vi "DAQ state machine with subvi.vi"() -> ()   [LabVIEW 2017]
uses:
  <vilib>/OPCUA/controls/Write Status.ctl
  <vilib>/OPCUA/controls/NodeId.ctl
  <vilib>/OPCUA/NI OPC UA Client.lvlib
  <vilib>/OPCUA/client/Multiple Write Double.vi
  <vilib>/OPCUA/client/Multiple Write Bool.vi
  <vilib>/OPCUA/controls/Subscription ID.ctl
  <vilib>/OPCUA/controls/OPC UA StatusCode.ctl
  <vilib>/OPCUA/controls/OPC UA Client Refnum.ctl
  <vilib>/OPCUA/controls/Subscription Data Change.ctl
  <vilib>/OPCUA/controls/Data Type.ctl
  <vilib>/OPCUA/controls/NodeIds.ctl
panel:
  out "Number of Disconnections":u32
  out "Available Elements for Reading":i32
  out "DAQ?":bool
  out "error out":errorcluster
  in  "error in (no error)":errorcluster
  out "Connection Status":bool
  in  "Stop":bool
  in  "Disconnect":bool
  in  "Connect to Server":bool
  in  "Flow Data?":bool=TRUE
  in  "Power Output On":bool
  in  "CTAH Set Point":sgl format="%.1f"
  in  "Pump Frequency [Hz]":dbl min=0.0 max=45.0 step=0.10000000149011612 format="%.1f"
  in  "Desired Power [W]":dbl min=0.0 max=10000.0 step=1.0 format="%.1f"
  in  "TCHX Frequency [Hz]":dbl min=0.0 max=60.0 step=0.10000000149011612 format="%.1f"
  out "Frequency [Hz] 3":dbl(slide) scale=0.0..60.0
  out "Frequency [Hz]":dbl(knob) scale=0.0..45.0
  out "WT-67":dbl format="%.1f"
  out "WT-64":dbl format="%.1f"
  out "WT-62":dbl format="%.1f"
  out "WT-61":dbl format="%.1f"
  out "WT-42":dbl format="%.1f"
  out "WT-40":dbl format="%.1f"
  out "WT-35":dbl format="%.1f"
  out "WT-33":dbl format="%.1f"
  out "WT-31":dbl format="%.1f"
  out "WT-28":dbl format="%.1f"
  out "WT-26":dbl format="%.1f"
  out "WT-24":dbl format="%.1f"
  out "WT-22":dbl format="%.1f"
  out "WT-20":dbl format="%.1f"
  out "WT-13":dbl format="%.1f"
  out "WT-10":dbl format="%.1f"
  out "ST-14w":dbl format="%.1f"
  out "ST-14s":dbl format="%.1f"
  out "ST-14n":dbl format="%.1f"
  out "ST-14e":dbl format="%.1f"
  out "ST-13":dbl format="%.1f"
  out "ST-12sw":dbl format="%.1f"
  out "ST-12se":dbl format="%.1f"
  out "ST-12n":dbl format="%.1f"
  out "ST-11":dbl format="%.1f"
  out "ST-10":dbl format="%.1f"
  out "CX-114":dbl format="%.1f"
  out "CX-113":dbl format="%.1f"
  out "CX-112":dbl format="%.1f"
  out "CX-111":dbl format="%.1f"
  out "CX-104":dbl format="%.1f"
  out "CX-103":dbl format="%.1f"
  out "CX-102":dbl format="%.1f"
  out "CX-101":dbl format="%.1f"
  out "BT-66":dbl format="%.1f"
  out "BT-65":sgl format="%.1f"
  out "BT-63":dbl format="%.1f"
  out "BT-60":dbl format="%.1f"
  out "BT-43":dbl format="%.1f"
  out "BT-41":dbl format="%.1f"
  out "BT-34":dbl format="%.1f"
  out "BT-32":dbl format="%.1f"
  out "BT-30":dbl format="%.1f"
  out "BT-29":sgl format="%.1f"
  out "BT-27":dbl format="%.1f"
  out "BT-25":dbl format="%.1f"
  out "BT-23":dbl format="%.1f"
  out "BT-21":dbl format="%.1f"
  out "BT-12":dbl format="%.1f"
  out "BT-11":dbl format="%.1f"
  out "20001":dbl
  out "AT-02":dbl format="%.1f"
  out "AT-01":dbl format="%.1f"
  out "System Time":timestamp
  out "DRACS Flow\n\n\nFM-60 [kg/s]":dbl format="%.3f"
  out "Primary Flow\n\n\nFM-40 [kg/s]":dbl format="%.3f"
  out "Bypass Flow\n\n\nFM-30 [kg/s]":dbl format="%.3f"
  out "DHX Primary Flow\n\n\nFM-20 [kg/s]":dbl format="%.3f"
  out "Temperature":dbl
  out "Time Stamp 2":timestamp
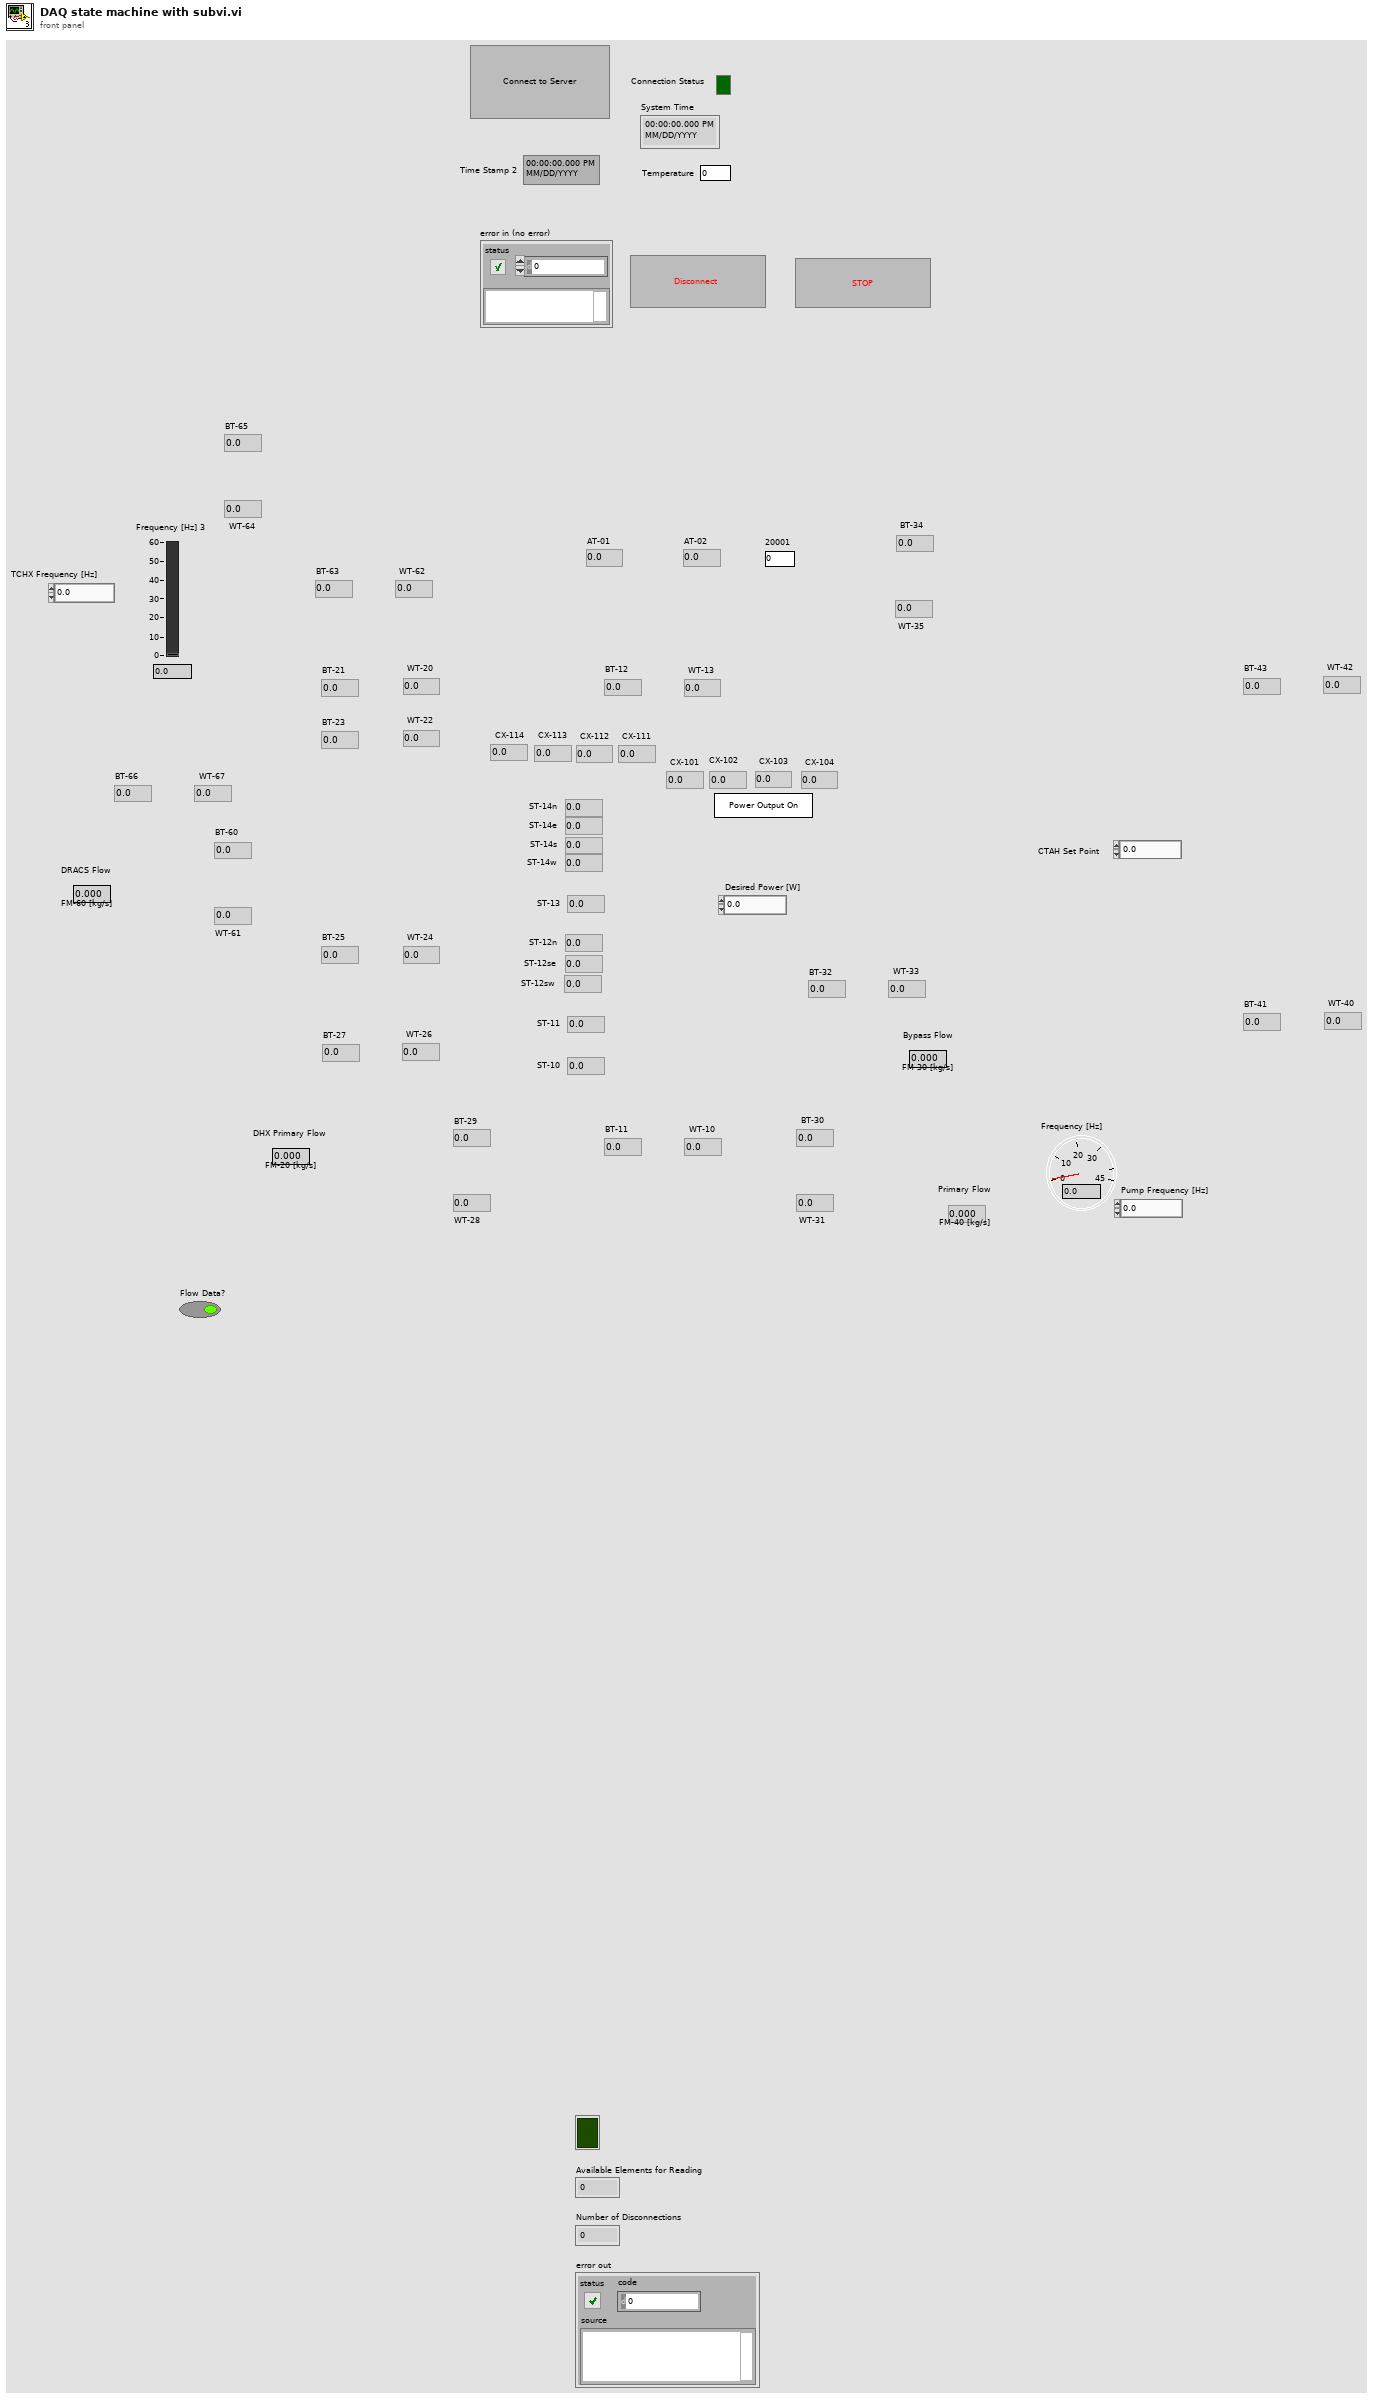
[diagram p1: front panel]
types:
  T1 = typedef "NodeId.ctl" = string
  T2 = typedef "Write Status.ctl" = u32
  T3 = cluster{"node ID":T1, "value":dbl, "timestamp (current time)":timestamp, "node status":T2}
  T4 = cluster{"node ID":T1, "value":bool, "timestamp (current time)":timestamp, "node status":T2}
  T5 = cluster{"message mode":enum16{"None", "Sign", "Sign and Encrypt"}, "security":enum16{"Basic256", "Basic128Rsa15"}}
  T6 = typedef "OPC UA Client Refnum.ctl" = refnum<k21>
  T7 = typedef "Subscription Data Change.ctl" = cluster{"node ID":T1, " value":variant, "timestamp":timestamp, "data type":T8, "status code":T9}
  T8 = typedef "Data Type.ctl" = u16
  T9 = typedef "OPC UA StatusCode.ctl" = u32
  T10 = cluster{"node ID":T1, "value":dbl, "timestamp (current time)":timestamp, "node status":T2}[]
  T11 = cluster{"node ID":T1, "value":bool, "timestamp (current time)":timestamp, "node status":T2}[]
  T12 = typedef "Subscription ID.ctl" = u32
  T13 = cluster{"OPC UA Data Change Event Registration Refnum":refnum<event-registration>, "OPC UA client refnum ":T6, "OPC UA Subscription Service Status":T9, "OPC UA Subscription ID":T12, "OPC UA Monitored Nodes":string[], "Connection Status":bool}
  T14 = typedef "NodeIds.ctl" = T1[]
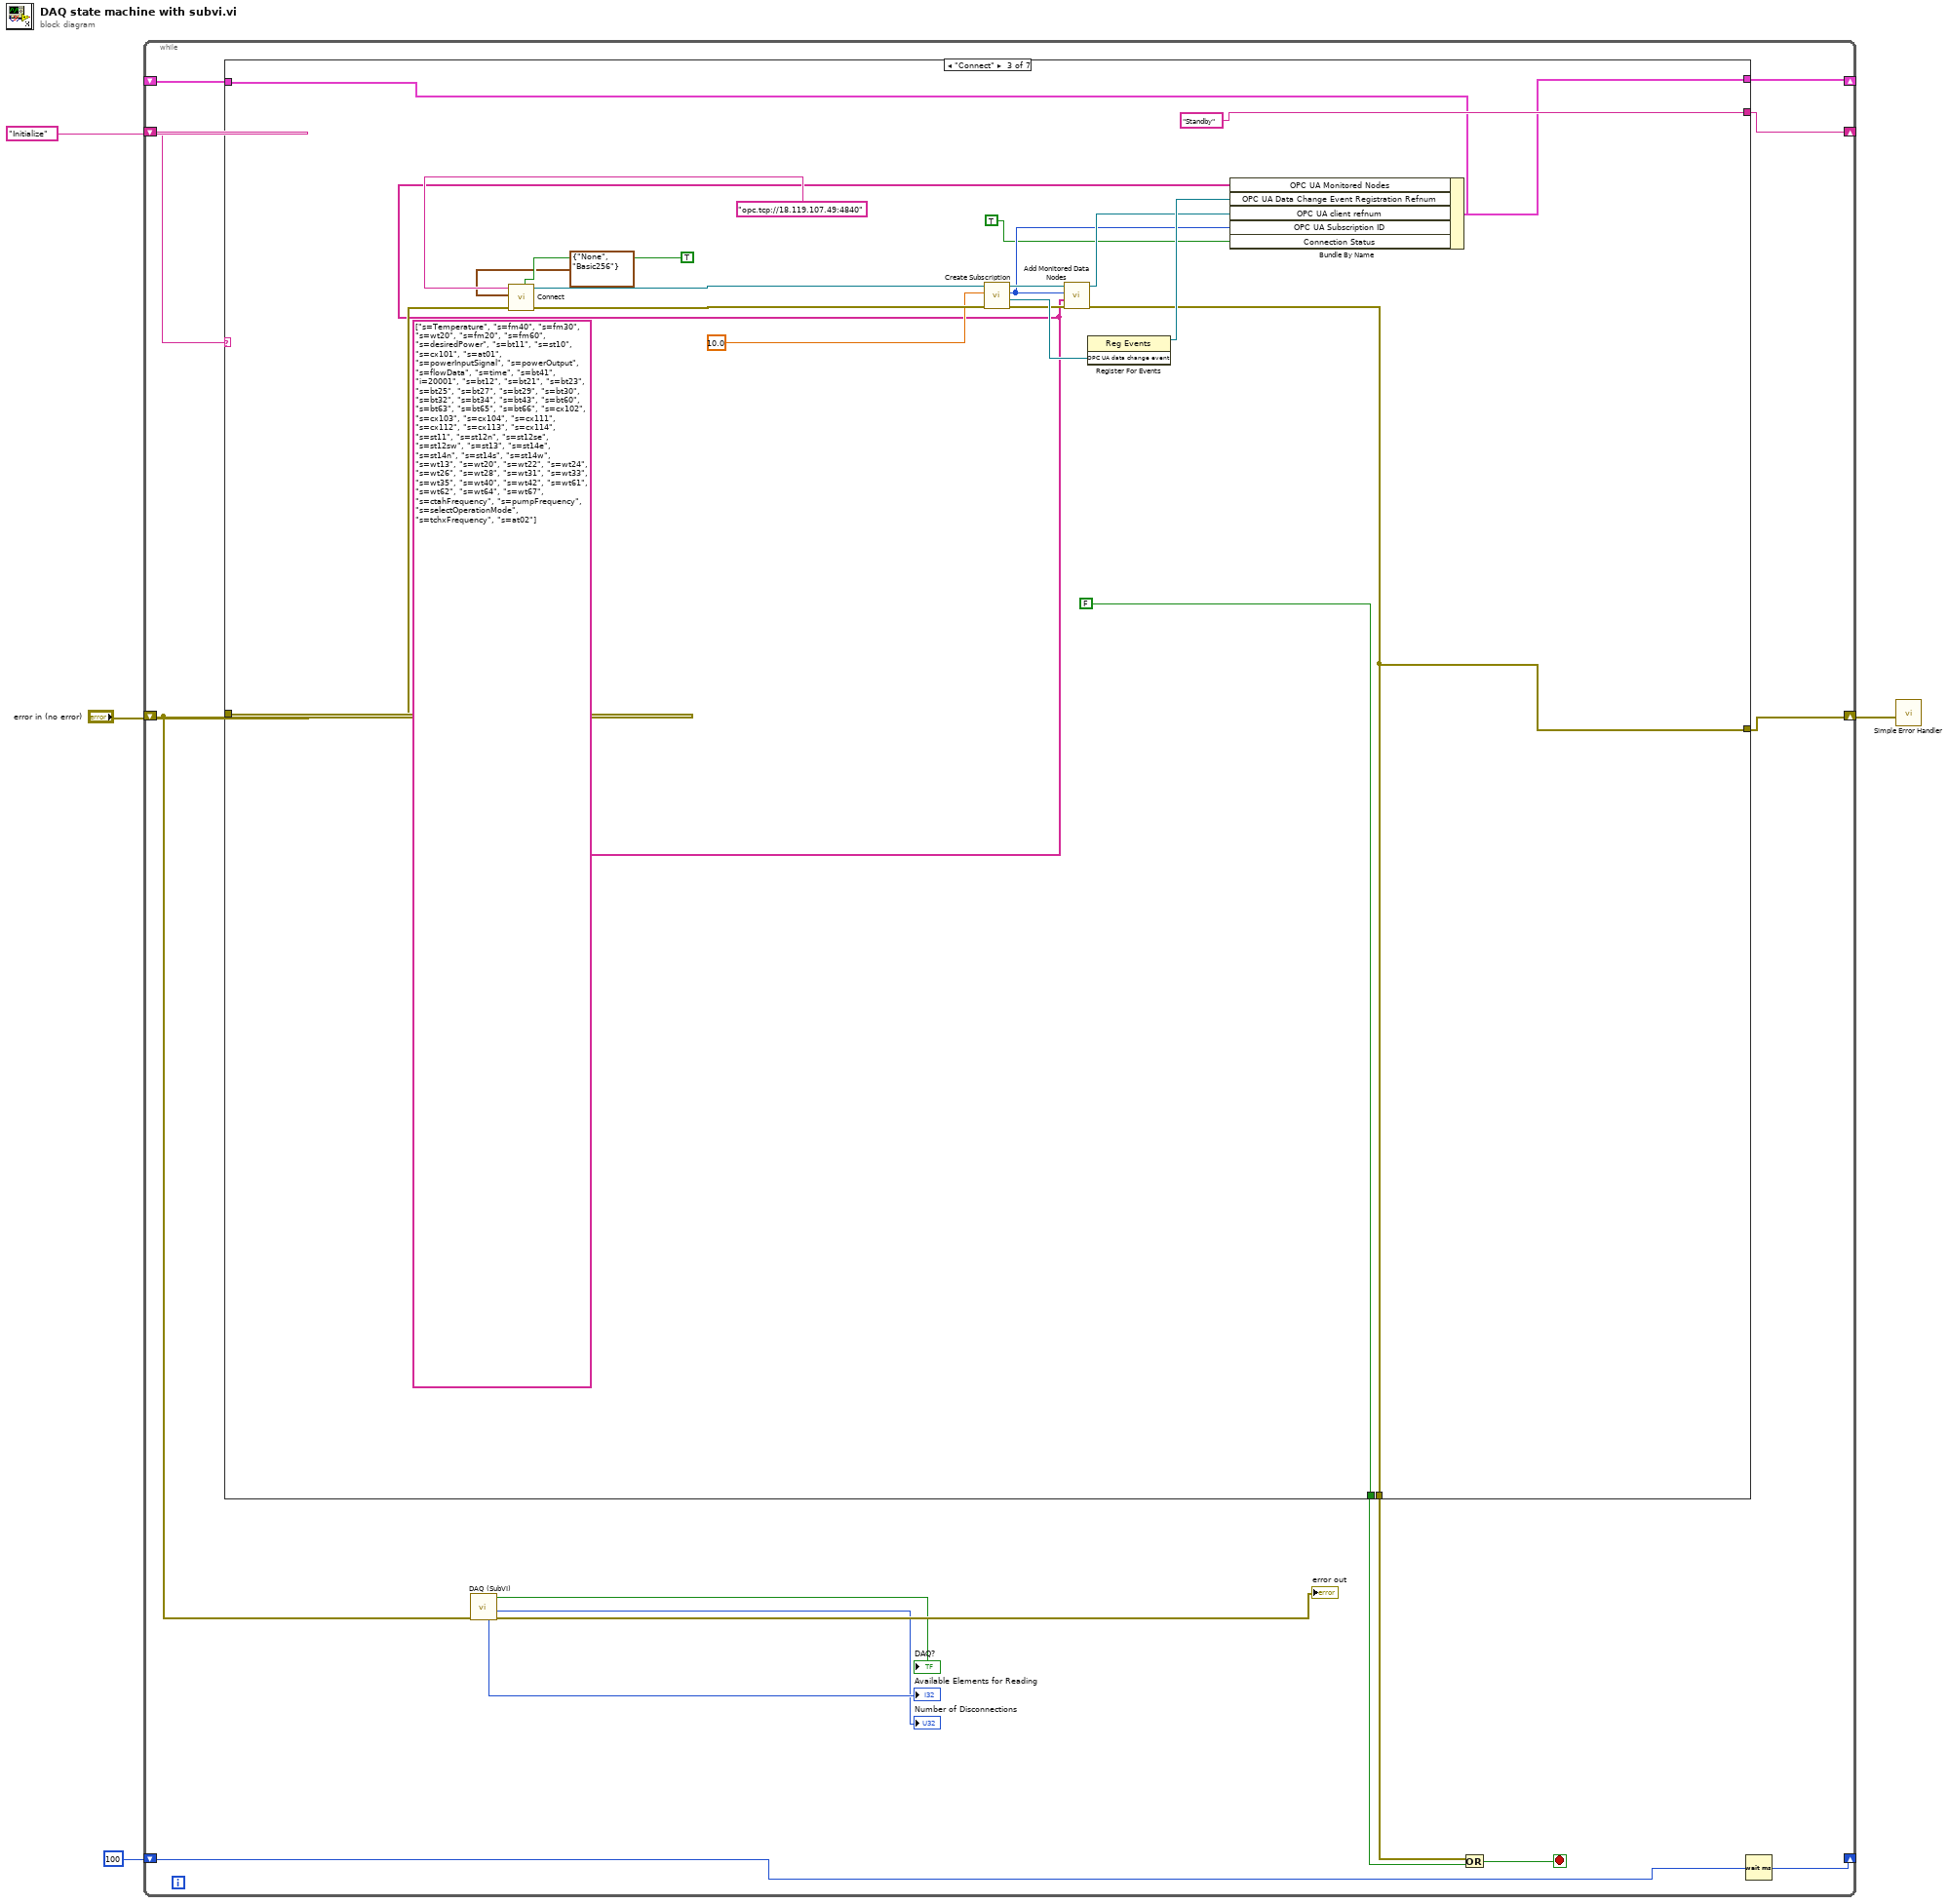
[diagram p0: block diagram]
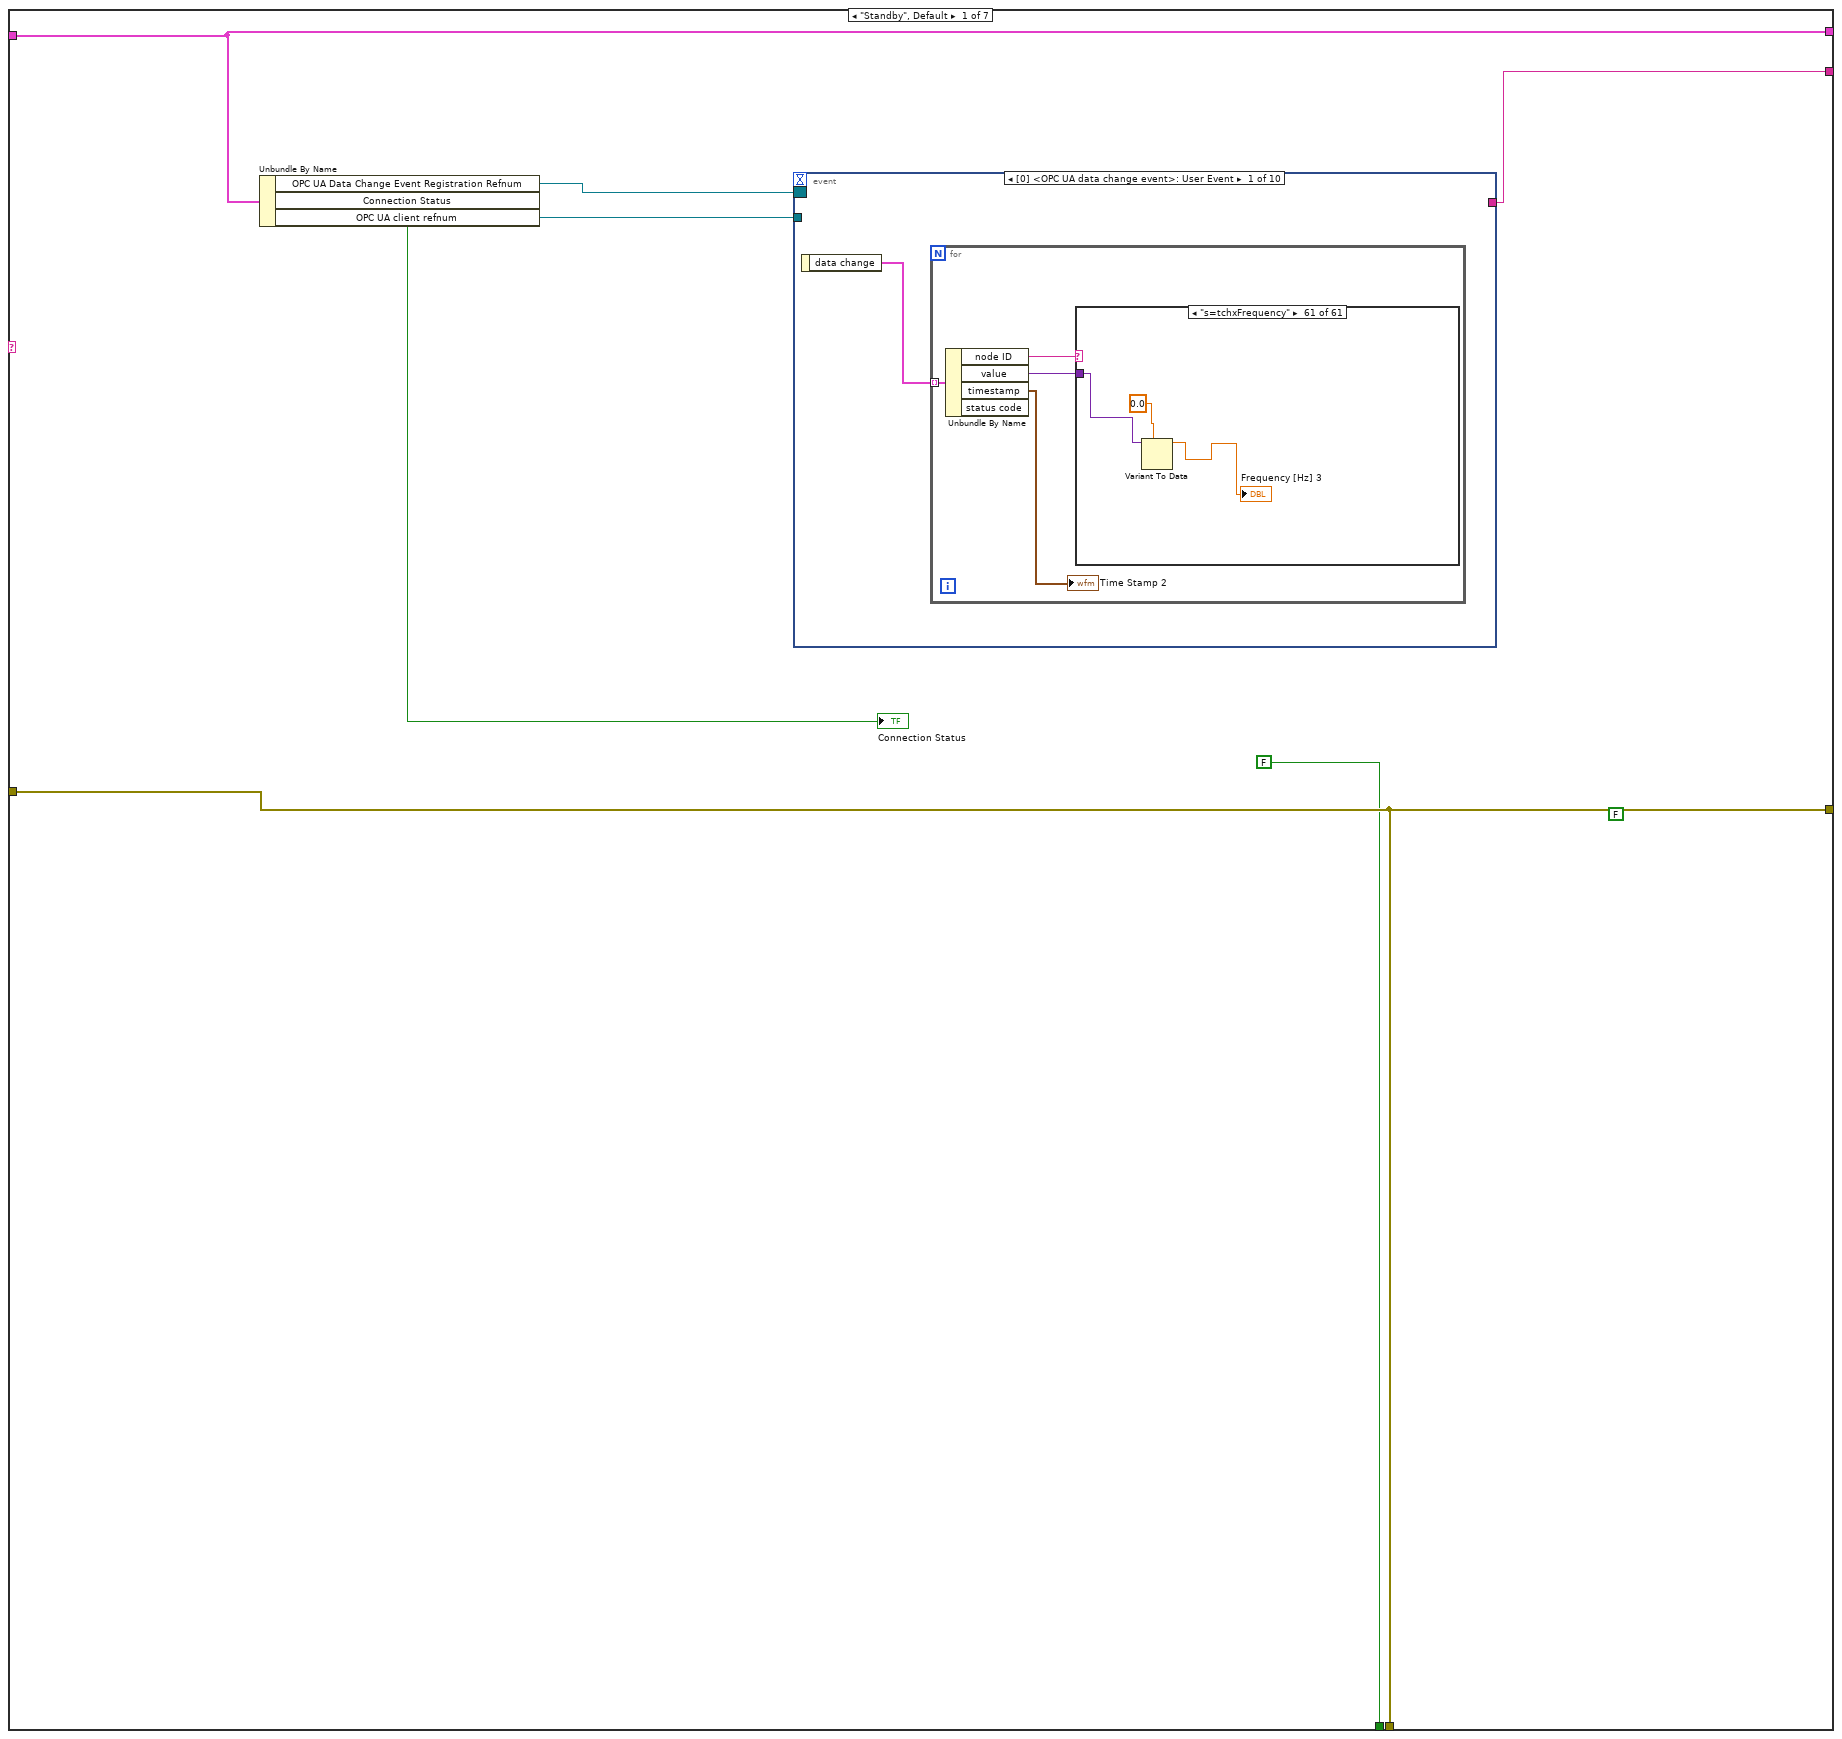
[diagram p2: hidden frame]
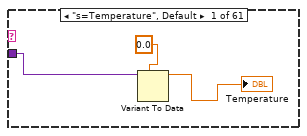
[diagram p3: hidden frame]
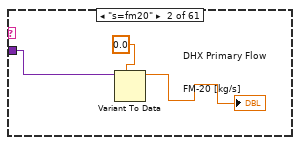
[diagram p4: hidden frame]
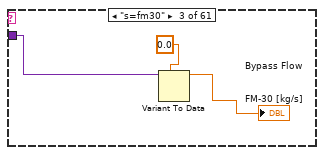
[diagram p5: hidden frame]
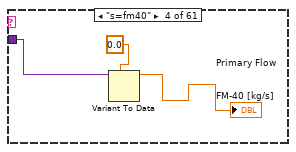
[diagram p6: hidden frame]
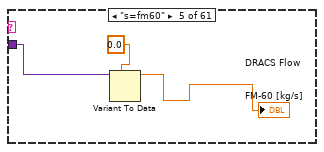
[diagram p7: hidden frame]
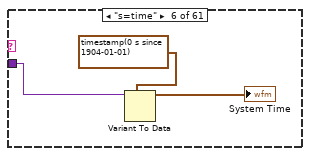
[diagram p8: hidden frame]
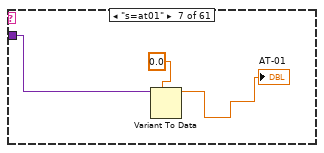
[diagram p9: hidden frame]
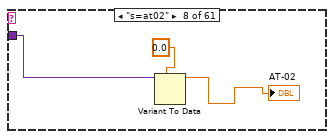
[diagram p10: hidden frame]
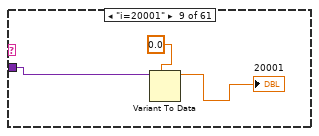
[diagram p11: hidden frame]
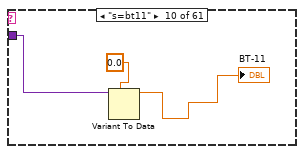
[diagram p12: hidden frame]
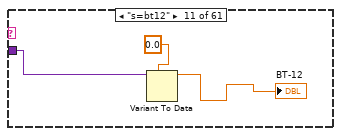
[diagram p13: hidden frame]
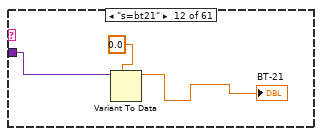
[diagram p14: hidden frame]
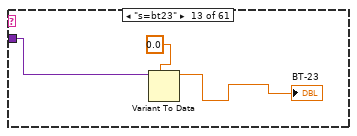
[diagram p15: hidden frame]
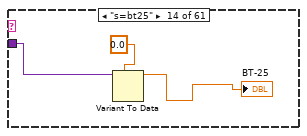
[diagram p16: hidden frame]
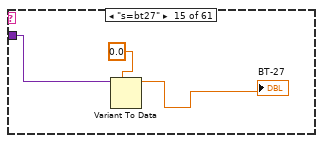
[diagram p17: hidden frame]
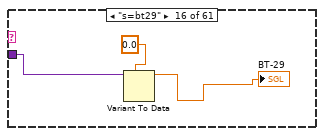
[diagram p18: hidden frame]
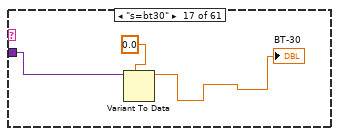
[diagram p19: hidden frame]
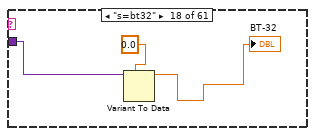
[diagram p20: hidden frame]
diagram:
  n1 = while {
    shift-right: [w15] -> _
    shift-left: _ -> [w16]
    shift-right: [w14] -> w3
    shift-left: "error in (no error)" -> [w5]
    shift-right: [w12] -> _
    shift-left: "Initialize" -> [w13]
    shift-right: [w10] -> _
    shift-left: u32 100 ("millisecond timer value") -> [w11]
    stop <- w18 stop-if-true
    n2 = case shown="\"Connect\"" w13 {
      tunnel: w5 -> [w22 w267 w285 w299 w318 w333 w342]
      tunnel: [w22 w267 w279 w299 w313 w328 w342] -> w19
      tunnel: [FALSE FALSE FALSE FALSE FALSE FALSE TRUE] -> w17
      tunnel: [w24 "Standby" "Standby" w300 "Standby" "Stop" "Initialize"] -> w12
      tunnel: [w23 w269 w278 w298 w311 w326 w341] -> w15
      tunnel: w16 -> [w23 w268 w281 w298 w312 w327 w341]
      tunnel: [w22 w267 w279 w299 w313 w328 w342] -> w14
      frame "Standby", Default {
        (unwired) FALSE
        n3 = Unbundle By Name(w23) -> ("OPC UA Data Change Event Registration Refnum"=w25:refnum<event-registration>, "Connection Status"=→"Connection Status":bool, "OPC UA client refnum"=w20:T6)
        n4 = event shown="[0] <OPC UA data change event>: User Event" {
          selector: w25 -> [_ _ _ _ _ _ _ _ _ _]
          dyn-events: _ -> [_ _ _ _ _ _ _ _ _ _]
          timeout: _ -> [_ _ _ _ _ _ _ _ _ _]
          tunnel: [_ _ _ _ _ _ _ "Connect" "Disconnect" "Stop Check"] -> w24
          tunnel: w20 -> [_ w215 w223 w235 w239 w247 w255 _ _ _]
          event User Event {
            n5 = event-data() -> ("data change"=w27:T7[])  [unwired: 1 in]
            n6 = for {
              tunnel: w27 -> [w30] mode=indexing
              n7 = Unbundle By Name(w30) -> ("node ID"=w29:T1, "value"=w28:variant, "timestamp"=→"Time Stamp 2":timestamp)  [unwired: 1 out]
              n8 = case shown="\"s=tchxFrequency\"" w29 {
                tunnel: w28 -> [w32 w36 w39 w42 w45 w49 w51 w53 w56 w60 w63 w66 w69 w72 w75 w78 w81 w84 w87 w90 w93 w96 w99 w102 w105 w108 w111 w114 w117 w120 w123 w126 w129 w132 w135 w138 w141 w144 w147 w150 w153 w156 w159 w162 w165 w168 w171 w174 w177 w180 w183 w186 w189 w192 w195 w198 w201 w204 w207 w210 w213]
                frame "s=Temperature", Default {
                  n9 = Variant To Data(type=0.0, Variant=w32) -> (data=→"Temperature":dbl)  [unwired: 1 in, 1 out]
                }
                frame "s=fm20" {
                  n10 = Variant To Data(type=0.0, Variant=w36) -> (data=→"DHX Primary Flow\n\n\nFM-20 [kg/s]":dbl)  [unwired: 1 in, 1 out]
                }
                frame "s=fm30" {
                  n11 = Variant To Data(type=0.0, Variant=w39) -> (data=→"Bypass Flow\n\n\nFM-30 [kg/s]":dbl)  [unwired: 1 in, 1 out]
                }
                frame "s=fm40" {
                  n12 = Variant To Data(type=0.0, Variant=w42) -> (data=→"Primary Flow\n\n\nFM-40 [kg/s]":dbl)  [unwired: 1 in, 1 out]
                }
                frame "s=fm60" {
                  n13 = Variant To Data(type=0.0, Variant=w45) -> (data=→"DRACS Flow\n\n\nFM-60 [kg/s]":dbl)  [unwired: 1 in, 1 out]
                }
                frame "s=time" {
                  n14 = Variant To Data(type=timestamp(0 s since 1904-01-01), Variant=w49) -> (data=→"System Time":timestamp)  [unwired: 1 in, 1 out]
                }
                frame "s=at01" {
                  n15 = Variant To Data(type=0.0, Variant=w51) -> (data=→"AT-01":dbl)  [unwired: 1 in, 1 out]
                }
                frame "s=at02" {
                  n16 = Variant To Data(type=0.0, Variant=w53) -> (data=→"AT-02":dbl)  [unwired: 1 in, 1 out]
                }
                frame "i=20001" {
                  n17 = Variant To Data(type=0.0, Variant=w56) -> (data=→"20001":dbl)  [unwired: 1 in, 1 out]
                }
                frame "s=bt11" {
                  n18 = Variant To Data(type=0.0, Variant=w60) -> (data=→"BT-11":dbl)  [unwired: 1 in, 1 out]
                }
                frame "s=bt12" {
                  n19 = Variant To Data(type=0.0, Variant=w63) -> (data=→"BT-12":dbl)  [unwired: 1 in, 1 out]
                }
                frame "s=bt21" {
                  n20 = Variant To Data(type=0.0, Variant=w66) -> (data=→"BT-21":dbl)  [unwired: 1 in, 1 out]
                }
                frame "s=bt23" {
                  n21 = Variant To Data(type=0.0, Variant=w69) -> (data=→"BT-23":dbl)  [unwired: 1 in, 1 out]
                }
                frame "s=bt25" {
                  n22 = Variant To Data(type=0.0, Variant=w72) -> (data=→"BT-25":dbl)  [unwired: 1 in, 1 out]
                }
                frame "s=bt27" {
                  n23 = Variant To Data(type=0.0, Variant=w75) -> (data=→"BT-27":dbl)  [unwired: 1 in, 1 out]
                }
                frame "s=bt29" {
                  n24 = Variant To Data(type=0.0, Variant=w78) -> (data=→"BT-29":dbl)  [unwired: 1 in, 1 out]
                }
                frame "s=bt30" {
                  n25 = Variant To Data(type=0.0, Variant=w81) -> (data=→"BT-30":dbl)  [unwired: 1 in, 1 out]
                }
                frame "s=bt32" {
                  n26 = Variant To Data(type=0.0, Variant=w84) -> (data=→"BT-32":dbl)  [unwired: 1 in, 1 out]
                }
                frame "s=bt34" {
                  n27 = Variant To Data(type=0.0, Variant=w87) -> (data=→"BT-34":dbl)  [unwired: 1 in, 1 out]
                }
                frame "s=bt41" {
                  n28 = Variant To Data(type=0.0, Variant=w90) -> (data=→"BT-41":dbl)  [unwired: 1 in, 1 out]
                }
                frame "s=bt43" {
                  n29 = Variant To Data(type=0.0, Variant=w93) -> (data=→"BT-43":dbl)  [unwired: 1 in, 1 out]
                }
                frame "s=bt60" {
                  n30 = Variant To Data(type=0.0, Variant=w96) -> (data=→"BT-60":dbl)  [unwired: 1 in, 1 out]
                }
                frame "s=bt63" {
                  n31 = Variant To Data(type=0.0, Variant=w99) -> (data=→"BT-63":dbl)  [unwired: 1 in, 1 out]
                }
                frame "s=bt65" {
                  n32 = Variant To Data(type=0.0, Variant=w102) -> (data=→"BT-65":dbl)  [unwired: 1 in, 1 out]
                }
                frame "s=bt66" {
                  n33 = Variant To Data(type=0.0, Variant=w105) -> (data=→"BT-66":dbl)  [unwired: 1 in, 1 out]
                }
                frame "s=cx101" {
                  n34 = Variant To Data(type=0.0, Variant=w108) -> (data=→"CX-101":dbl)  [unwired: 1 in, 1 out]
                }
                frame "s=cx102" {
                  n35 = Variant To Data(type=0.0, Variant=w111) -> (data=→"CX-102":dbl)  [unwired: 1 in, 1 out]
                }
                frame "s=cx103" {
                  n36 = Variant To Data(type=0.0, Variant=w114) -> (data=→"CX-103":dbl)  [unwired: 1 in, 1 out]
                }
                frame "s=cx104" {
                  n37 = Variant To Data(type=0.0, Variant=w117) -> (data=→"CX-104":dbl)  [unwired: 1 in, 1 out]
                }
                frame "s=cx111" {
                  n38 = Variant To Data(type=0.0, Variant=w120) -> (data=→"CX-111":dbl)  [unwired: 1 in, 1 out]
                }
                frame "s=cx112" {
                  n39 = Variant To Data(type=0.0, Variant=w123) -> (data=→"CX-112":dbl)  [unwired: 1 in, 1 out]
                }
                frame "s=cx113" {
                  n40 = Variant To Data(type=0.0, Variant=w126) -> (data=→"CX-113":dbl)  [unwired: 1 in, 1 out]
                }
                frame "s=cx114" {
                  n41 = Variant To Data(type=0.0, Variant=w129) -> (data=→"CX-114":dbl)  [unwired: 1 in, 1 out]
                }
                frame "s=st10" {
                  n42 = Variant To Data(type=0.0, Variant=w132) -> (data=→"ST-10":dbl)  [unwired: 1 in, 1 out]
                }
                frame "s=st11" {
                  n43 = Variant To Data(type=0.0, Variant=w135) -> (data=→"ST-11":dbl)  [unwired: 1 in, 1 out]
                }
                frame "s=st12n" {
                  n44 = Variant To Data(type=0.0, Variant=w138) -> (data=→"ST-12n":dbl)  [unwired: 1 in, 1 out]
                }
                frame "s=st12se" {
                  n45 = Variant To Data(type=0.0, Variant=w141) -> (data=→"ST-12se":dbl)  [unwired: 1 in, 1 out]
                }
                frame "s=st12sw" {
                  n46 = Variant To Data(type=0.0, Variant=w144) -> (data=→"ST-12sw":dbl)  [unwired: 1 in, 1 out]
                }
                frame "s=st13" {
                  n47 = Variant To Data(type=0.0, Variant=w147) -> (data=→"ST-13":dbl)  [unwired: 1 in, 1 out]
                }
                frame "s=st14e" {
                  n48 = Variant To Data(type=0.0, Variant=w150) -> (data=→"ST-14e":dbl)  [unwired: 1 in, 1 out]
                }
                frame "s=st14n" {
                  n49 = Variant To Data(type=0.0, Variant=w153) -> (data=→"ST-14n":dbl)  [unwired: 1 in, 1 out]
                }
                frame "s=st14s" {
                  n50 = Variant To Data(type=0.0, Variant=w156) -> (data=→"ST-14s":dbl)  [unwired: 1 in, 1 out]
                }
                frame "s=st14w" {
                  n51 = Variant To Data(type=0.0, Variant=w159) -> (data=→"ST-14w":dbl)  [unwired: 1 in, 1 out]
                }
                frame "s=wt10" {
                  n52 = Variant To Data(type=0.0, Variant=w162) -> (data=→"WT-10":dbl)  [unwired: 1 in, 1 out]
                }
                frame "s=wt13" {
                  n53 = Variant To Data(type=0.0, Variant=w165) -> (data=→"WT-13":dbl)  [unwired: 1 in, 1 out]
                }
                frame "s=wt20" {
                  n54 = Variant To Data(type=0.0, Variant=w168) -> (data=→"WT-20":dbl)  [unwired: 1 in, 1 out]
                }
                frame "s=wt22" {
                  n55 = Variant To Data(type=0.0, Variant=w171) -> (data=→"WT-22":dbl)  [unwired: 1 in, 1 out]
                }
                frame "s=wt24" {
                  n56 = Variant To Data(type=0.0, Variant=w174) -> (data=→"WT-24":dbl)  [unwired: 1 in, 1 out]
                }
                frame "s=wt26" {
                  n57 = Variant To Data(type=0.0, Variant=w177) -> (data=→"WT-26":dbl)  [unwired: 1 in, 1 out]
                }
                frame "s=wt28" {
                  n58 = Variant To Data(type=0.0, Variant=w180) -> (data=→"WT-28":dbl)  [unwired: 1 in, 1 out]
                }
                frame "s=wt31" {
                  n59 = Variant To Data(type=0.0, Variant=w183) -> (data=→"WT-31":dbl)  [unwired: 1 in, 1 out]
                }
                frame "s=wt33" {
                  n60 = Variant To Data(type=0.0, Variant=w186) -> (data=→"WT-33":dbl)  [unwired: 1 in, 1 out]
                }
                frame "s=wt35" {
                  n61 = Variant To Data(type=0.0, Variant=w189) -> (data=→"WT-35":dbl)  [unwired: 1 in, 1 out]
                }
                frame "s=wt40" {
                  n62 = Variant To Data(type=0.0, Variant=w192) -> (data=→"WT-40":dbl)  [unwired: 1 in, 1 out]
                }
                frame "s=wt42" {
                  n63 = Variant To Data(type=0.0, Variant=w195) -> (data=→"WT-42":dbl)  [unwired: 1 in, 1 out]
                }
                frame "s=wt61" {
                  n64 = Variant To Data(type=0.0, Variant=w198) -> (data=→"WT-61":dbl)  [unwired: 1 in, 1 out]
                }
                frame "s=wt62" {
                  n65 = Variant To Data(type=0.0, Variant=w201) -> (data=→"WT-62":dbl)  [unwired: 1 in, 1 out]
                }
                frame "s=wt64" {
                  n66 = Variant To Data(type=0.0, Variant=w204) -> (data=→"WT-64":dbl)  [unwired: 1 in, 1 out]
                }
                frame "s=wt67" {
                  n67 = Variant To Data(type=0.0, Variant=w207) -> (data=→"WT-67":dbl)  [unwired: 1 in, 1 out]
                }
                frame "s=pumpFrequency" {
                  n68 = Variant To Data(type=0.0, Variant=w210) -> (data=→"Frequency [Hz]":dbl)  [unwired: 1 in, 1 out]
                }
                frame "s=tchxFrequency" {
                  n69 = Variant To Data(type=0.0, Variant=w213) -> (data=→"Frequency [Hz] 3":dbl)  [unwired: 1 in, 1 out]
                }
              }
            }
          }
          event "TCHX Frequency [Hz]": Value Change {
            w222 = T2 0 items=["Good"=0, "Uncertain_InitialValue"=1083310080, "Uncertain_LastUsableValue"=1083179008, "Uncertain_SensorNotAccurate"=1083375616, "Uncertain_EngineeringUnitsExceeded"=1083441152, "Bad_NoCommunication"=2150694912, "Bad_NotReadable"=2151284736, "Bad_NotWritable"=2151350272, "Bad_OutOfRange"=2151415808, "Bad_WaitingForInitialData"=2150760448] ("node status")
            n70 = event-data() -> ()  [unwired: 1 in, 6 out]
            n71 = Bundle By Name(cluster=T3 {"node ID"="", "value"=0.0, "timestamp (current time)"=timestamp(0 s since 1904-01-01), "node status"=0} ("request"), "node ID"="s=tchxFrequency", "value"="TCHX Frequency [Hz]", "timestamp (current time)"=timestamp(0 s since 1904-01-01), "node status"=w222) -> (w219:T3)
            n72 = Build Array(w219) -> (w217:T10)
            n73 = call-poly <vilib>:"Multiple Write.vi"("requests"=w217, "OPC UA client refnum in"=w215) -> ()  [unwired: 6 in, 4 out]
          }
          event "Desired Power [W]": Value Change {
            w230 = T2 0 items=["Good"=0, "Uncertain_InitialValue"=1083310080, "Uncertain_LastUsableValue"=1083179008, "Uncertain_SensorNotAccurate"=1083375616, "Uncertain_EngineeringUnitsExceeded"=1083441152, "Bad_NoCommunication"=2150694912, "Bad_NotReadable"=2151284736, "Bad_NotWritable"=2151350272, "Bad_OutOfRange"=2151415808, "Bad_WaitingForInitialData"=2150760448] ("node status")
            n74 = event-data() -> ()  [unwired: 1 in, 6 out]
            n75 = Bundle By Name(cluster=T3 {"node ID"="", "value"=0.0, "timestamp (current time)"=timestamp(0 s since 1904-01-01), "node status"=0} ("request"), "node ID"="s=desiredPower", "value"="Desired Power [W]", "timestamp (current time)"=timestamp(0 s since 1904-01-01), "node status"=w230) -> (w227:T3)
            n76 = Build Array(w227) -> (w225:T10)
            n77 = call-poly <vilib>:"Multiple Write.vi"("requests"=w225, "OPC UA client refnum in"=w223) -> ()  [unwired: 6 in, 4 out]
          }
          event "Pump Frequency [Hz]": Value Change {
            w238 = T2 0 items=["Good"=0, "Uncertain_InitialValue"=1083310080, "Uncertain_LastUsableValue"=1083179008, "Uncertain_SensorNotAccurate"=1083375616, "Uncertain_EngineeringUnitsExceeded"=1083441152, "Bad_NoCommunication"=2150694912, "Bad_NotReadable"=2151284736, "Bad_NotWritable"=2151350272, "Bad_OutOfRange"=2151415808, "Bad_WaitingForInitialData"=2150760448] ("node status")
            n78 = event-data() -> ()  [unwired: 1 in, 6 out]
            n79 = Bundle By Name(cluster=T3 {"node ID"="", "value"=0.0, "timestamp (current time)"=timestamp(0 s since 1904-01-01), "node status"=0} ("request"), "node ID"="s=pumpFrequency", "value"="Pump Frequency [Hz]", "timestamp (current time)"=timestamp(0 s since 1904-01-01), "node status"=w238) -> (w233:T3)
            n80 = Build Array(w233) -> (w231:T10)
            n81 = call-poly <vilib>:"Multiple Write.vi"("requests"=w231, "OPC UA client refnum in"=w235) -> ()  [unwired: 6 in, 4 out]
          }
          event "CTAH Set Point": Value Change {
            w246 = T2 0 items=["Good"=0, "Uncertain_InitialValue"=1083310080, "Uncertain_LastUsableValue"=1083179008, "Uncertain_SensorNotAccurate"=1083375616, "Uncertain_EngineeringUnitsExceeded"=1083441152, "Bad_NoCommunication"=2150694912, "Bad_NotReadable"=2151284736, "Bad_NotWritable"=2151350272, "Bad_OutOfRange"=2151415808, "Bad_WaitingForInitialData"=2150760448] ("node status")
            n82 = event-data() -> ()  [unwired: 1 in, 6 out]
            n83 = Bundle By Name(cluster=T3 {"node ID"="", "value"=0.0, "timestamp (current time)"=timestamp(0 s since 1904-01-01), "node status"=0} ("request"), "node ID"="s=ctahSetPoint", "value"="CTAH Set Point", "timestamp (current time)"=timestamp(0 s since 1904-01-01), "node status"=w246) -> (w243:T3)
            n84 = Build Array(w243) -> (w241:T10)
            n85 = call-poly <vilib>:"Multiple Write.vi"("requests"=w241, "OPC UA client refnum in"=w239) -> ()  [unwired: 6 in, 4 out]
          }
          event "Power Output On": Value Change {
            w253 = T2 0 items=["Good"=0, "Uncertain_InitialValue"=1083310080, "Uncertain_LastUsableValue"=1083179008, "Uncertain_SensorNotAccurate"=1083375616, "Uncertain_EngineeringUnitsExceeded"=1083441152, "Bad_NoCommunication"=2150694912, "Bad_NotReadable"=2151284736, "Bad_NotWritable"=2151350272, "Bad_OutOfRange"=2151415808, "Bad_WaitingForInitialData"=2150760448] ("node status")
            n86 = event-data() -> ()  [unwired: 1 in, 6 out]
            n87 = Bundle By Name(cluster=T4 {"node ID"="", "value"=FALSE, "timestamp (current time)"=timestamp(0 s since 1904-01-01), "node status"=0} ("request"), "node ID"="s=powerOutputOn", "value"="Power Output On", "timestamp (current time)"=timestamp(0 s since 1904-01-01), "node status"=w253) -> (w250:T4)
            n88 = Build Array(w250) -> (w249:T11)
            n89 = call-poly <vilib>:"Multiple Write.vi"("requests"=w249, "OPC UA client refnum in"=w247) -> ()  [unwired: 6 in, 4 out]
          }
          event "Flow Data?": Value Change {
            w261 = T2 0 items=["Good"=0, "Uncertain_InitialValue"=1083310080, "Uncertain_LastUsableValue"=1083179008, "Uncertain_SensorNotAccurate"=1083375616, "Uncertain_EngineeringUnitsExceeded"=1083441152, "Bad_NoCommunication"=2150694912, "Bad_NotReadable"=2151284736, "Bad_NotWritable"=2151350272, "Bad_OutOfRange"=2151415808, "Bad_WaitingForInitialData"=2150760448] ("node status")
            n90 = event-data() -> ()  [unwired: 1 in, 6 out]
            n91 = Bundle By Name(cluster=T4 {"node ID"="", "value"=FALSE, "timestamp (current time)"=timestamp(0 s since 1904-01-01), "node status"=0} ("request"), "node ID"="s=activatePump", "value"="Flow Data?", "timestamp (current time)"=timestamp(0 s since 1904-01-01), "node status"=w261) -> (w258:T4)
            n92 = Build Array(w258) -> (w257:T11)
            n93 = call-poly <vilib>:"Multiple Write.vi"("requests"=w257, "OPC UA client refnum in"=w255) -> ()  [unwired: 6 in, 4 out]
          }
          event "Connect to Server": Value Change {
            n94 = event-data() -> ()  [unwired: 1 in, 6 out]
          }
          event "Disconnect": Value Change {
            n95 = event-data() -> ()  [unwired: 1 in, 6 out]
          }
          event "Stop": Value Change {
            n96 = event-data() -> ()  [unwired: 1 in, 6 out]
          }
        }
      }
      frame "Initialize" {
        w270 = FALSE  # Connection Status
        w271 = string[] []  # OPC UA Monitored Nodes
        w272 = T12 0  # OPC UA Subscription ID
        w273 = T9 0 items=["Good"=0, "Good_SubscriptionTransferred"=2949120, "Good_CompletesAsynchronously"=3014656, "Good_Overload"=3080192, "Good_Clamped"=3145728, "Good_LocalOverride"=9830400, "Good_EntryInserted"=10616832, "Good_EntryReplaced"=10682368, "Good_NoData"=10813440, "Good_MoreData"=10878976, "Good_CommunicationEvent"=10944512, "Good_ShutdownEvent"=11010048, "Good_CallAgain"=11075584, "Good_NonCriticalTimeout"=11141120, "Good_ResultsMayBeIncomplete"=12189696, "Good_DataIgnored"=14221312, "Uncertain"=1073741824, "Uncertain_ReferenceOutOfServer"=1080819712, "Uncertain_NoCommunicationLastUsableValue"=1083113472, "Uncertain_LastUsableValue"=1083179008, "Uncertain_SubstituteValue"=1083244544, "Uncertain_InitialValue"=1083310080, "Uncertain_SensorNotAccurate"=1083375616, "Uncertain_EngineeringUnitsExceeded"=1083441152, "Uncertain_SubNormal"=1083506688, "Uncertain_DataSubNormal"=1084489728, "Uncertain_ReferenceNotDeleted"=1086062592, "Uncertain_NotAllNodesAvailable"=1086324736, "Bad"=2147483648, "Bad_UnexpectedError"=2147549184, "Bad_InternalError"=2147614720, "Bad_OutOfMemory"=2147680256, "Bad_ResourceUnavailable"=2147745792, "Bad_CommunicationError"=2147811328, "Bad_EncodingError"=2147876864, "Bad_DecodingError"=2147942400, "Bad_EncodingLimitsExceeded"=2148007936, "Bad_UnknownResponse"=2148073472, "Bad_Timeout"=2148139008, "Bad_ServiceUnsupported"=2148204544, "Bad_Shutdown"=2148270080, "Bad_ServerNotConnected"=2148335616, "Bad_ServerHalted"=2148401152, "Bad_NothingToDo"=2148466688, "Bad_TooManyOperations"=2148532224, "Bad_DataTypeIdUnknown"=2148597760, "Bad_CertificateInvalid"=2148663296, "Bad_SecurityChecksFailed"=2148728832, "Bad_CertificateTimeInvalid"=2148794368, "Bad_CertificateIssuerTimeInvalid"=2148859904, "Bad_CertificateHostNameInvalid"=2148925440, "Bad_CertificateUriInvalid"=2148990976, "Bad_CertificateUseNotAllowed"=2149056512, "Bad_CertificateIssuerUseNotAllowed"=2149122048, "Bad_CertificateUntrusted"=2149187584, "Bad_CertificateRevocationUnknown"=2149253120, "Bad_CertificateIssuerRevocationUnknown"=2149318656, "Bad_CertificateRevoked"=2149384192, "Bad_CertificateIssuerRevoked"=2149449728, "Bad_UserAccessDenied"=2149515264, "Bad_IdentityTokenInvalid"=2149580800, "Bad_IdentityTokenRejected"=2149646336, "Bad_SecureChannelIdInvalid"=2149711872, "Bad_InvalidTimestamp"=2149777408, "Bad_NonceInvalid"=2149842944, "Bad_SessionIdInvalid"=2149908480, "Bad_SessionClosed"=2149974016, "Bad_SessionNotActivated"=2150039552, "Bad_SubscriptionIdInvalid"=2150105088, "Bad_RequestHeaderInvalid"=2150236160, "Bad_TimestampsToReturnInvalid"=2150301696, "Bad_RequestCancelledByClient"=2150367232, "Bad_NoCommunication"=2150694912, "Bad_WaitingForInitialData"=2150760448, "Bad_NodeIdInvalid"=2150825984, "Bad_NodeIdUnknown"=2150891520, "Bad_AttributeIdInvalid"=2150957056, "Bad_IndexRangeInvalid"=2151022592, "Bad_IndexRangeNoData"=2151088128, "Bad_DataEncodingInvalid"=2151153664, "Bad_DataEncodingUnsupported"=2151219200, "Bad_NotReadable"=2151284736, "Bad_NotWritable"=2151350272, "Bad_OutOfRange"=2151415808, "Bad_NotSupported"=2151481344, "Bad_NotFound"=2151546880, "Bad_ObjectDeleted"=2151612416, "Bad_NotImplemented"=2151677952, "Bad_MonitoringModeInvalid"=2151743488, "Bad_MonitoredItemIdInvalid"=2151809024, "Bad_MonitoredItemFilterInvalid"=2151874560, "Bad_MonitoredItemFilterUnsupported"=2151940096, "Bad_FilterNotAllowed"=2152005632, "Bad_StructureMissing"=2152071168, "Bad_EventFilterInvalid"=2152136704, "Bad_ContentFilterInvalid"=2152202240, "Bad_FilterOperandInvalid"=2152267776, "Bad_ContinuationPointInvalid"=2152333312, "Bad_NoContinuationPoints"=2152398848, "Bad_ReferenceTypeIdInvalid"=2152464384, "Bad_BrowseDirectionInvalid"=2152529920, "Bad_NodeNotInView"=2152595456, "Bad_ServerUriInvalid"=2152660992, "Bad_ServerNameMissing"=2152726528, "Bad_DiscoveryUrlMissing"=2152792064, "Bad_SempahoreFileMissing"=2152857600, "Bad_RequestTypeInvalid"=2152923136, "Bad_SecurityModeRejected"=2152988672, "Bad_SecurityPolicyRejected"=2153054208, "Bad_TooManySessions"=2153119744, "Bad_UserSignatureInvalid"=2153185280, "Bad_ApplicationSignatureInvalid"=2153250816, "Bad_NoValidCertificates"=2153316352, "Bad_RequestCancelledByRequest"=2153381888, "Bad_ParentNodeIdInvalid"=2153447424, "Bad_ReferenceNotAllowed"=2153512960, "Bad_NodeIdRejected"=2153578496, "Bad_NodeIdExists"=2153644032, "Bad_NodeClassInvalid"=2153709568, "Bad_BrowseNameInvalid"=2153775104, "Bad_BrowseNameDuplicated"=2153840640, "Bad_NodeAttributesInvalid"=2153906176, "Bad_TypeDefinitionInvalid"=2153971712, "Bad_SourceNodeIdInvalid"=2154037248, "Bad_TargetNodeIdInvalid"=2154102784, "Bad_DuplicateReferenceNotAllowed"=2154168320, "Bad_InvalidSelfReference"=2154233856, "Bad_ReferenceLocalOnly"=2154299392, "Bad_NoDeleteRights"=2154364928, "Bad_ServerIndexInvalid"=2154430464, "Bad_ViewIdUnknown"=2154496000, "Bad_TooManyMatches"=2154627072, "Bad_QueryTooComplex"=2154692608, "Bad_NoMatch"=2154758144, "Bad_MaxAgeInvalid"=2154823680, "Bad_HistoryOperationInvalid"=2154889216, "Bad_HistoryOperationUnsupported"=2154954752, "Bad_WriteNotSupported"=2155020288, "Bad_TypeMismatch"=2155085824, "Bad_MethodInvalid"=2155151360, "Bad_ArgumentsMissing"=2155216896, "Bad_TooManySubscriptions"=2155282432, "Bad_TooManyPublishRequests"=2155347968, "Bad_NoSubscription"=2155413504, "Bad_SequenceNumberUnknown"=2155479040, "Bad_MessageNotAvailable"=2155544576, "Bad_InsufficientClientProfile"=2155610112, "Bad_TcpServerTooBusy"=2155675648, "Bad_TcpMessageTypeInvalid"=2155741184, "Bad_TcpSecureChannelUnknown"=2155806720, "Bad_TcpMessageTooLarge"=2155872256, "Bad_TcpNotEnoughResources"=2155937792, "Bad_TcpInternalError"=2156003328, "Bad_TcpEndpointUrlInvalid"=2156068864, "Bad_RequestInterrupted"=2156134400, "Bad_RequestTimeout"=2156199936, "Bad_SecureChannelClosed"=2156265472, "Bad_SecureChannelTokenUnknown"=2156331008, "Bad_SequenceNumberInvalid"=2156396544, "Bad_ConfigurationError"=2156462080, "Bad_NotConnected"=2156527616, "Bad_DeviceFailure"=2156593152, "Bad_SensorFailure"=2156658688, "Bad_OutOfService"=2156724224, "Bad_DeadbandFilterInvalid"=2156789760, "Bad_RefreshInProgress"=2157379584, "Bad_ConditionAlreadyDisabled"=2157445120, "Bad_ConditionDisabled"=2157510656, "Bad_EventIdUnknown"=2157576192, "Bad_NoData"=2157641728, "Bad_DataLost"=2157772800, "Bad_DataUnavailable"=2157838336, "Bad_EntryExists"=2157903872, "Bad_NoEntryExists"=2157969408, "Bad_TimestampNotSupported"=2158034944, "Bad_InvalidArgument"=2158690304, "Bad_ConnectionRejected"=2158755840, "Bad_Disconnect"=2158821376, "Bad_ConnectionClosed"=2158886912, "Bad_InvalidState"=2158952448, "Bad_EndOfStream"=2159017984, "Bad_NoDataAvailable"=2159083520, "Bad_WaitingForResponse"=2159149056, "Bad_OperationAbandoned"=2159214592, "Bad_ExpectedStreamToBlock"=2159280128, "Bad_WouldBlock"=2159345664, "Bad_SyntaxError"=2159411200, "Bad_MaxConnectionsReached"=2159476736, "Bad_RequestTooLarge"=2159542272, "Bad_ResponseTooLarge"=2159607808, "Bad_EventNotAcknowledgeable"=2159738880, "Bad_InvalidTimestampArgument"=2159869952, "Bad_ProtocolVersionUnsupported"=2159935488, "Bad_StateNotActive"=2160001024, "Bad_FilterOperatorInvalid"=2160132096, "Bad_FilterOperatorUnsupported"=2160197632, "Bad_FilterOperandCountMismatch"=2160263168, "Bad_FilterElementInvalid"=2160328704, "Bad_FilterLiteralInvalid"=2160394240, "Bad_IdentityChangeNotSupported"=2160459776, "Bad_NotTypeDefinition"=2160590848, "Bad_ViewTimestampInvalid"=2160656384, "Bad_ViewParameterMismatch"=2160721920, "Bad_ViewVersionInvalid"=2160787456, "Bad_ConditionAlreadyEnabled"=2160852992, "Bad_DialogNotActive"=2160918528, "Bad_DialogResponseInvalid"=2160984064, "Bad_ConditionBranchAlreadyAcked"=2161049600, "Bad_ConditionBranchAlreadyConfirmed"=2161115136, "Bad_ConditionAlreadyShelved"=2161180672, "Bad_ConditionNotShelved"=2161246208, "Bad_ShelvingTimeOutOfRange"=2161311744, "Bad_AggregateListMismatch"=2161377280, "Bad_AggregateNotSupported"=2161442816, "Bad_AggregateInvalidInputs"=2161508352, "Bad_BoundNotFound"=2161573888, "Bad_BoundNotSupported"=2161639424, "Bad_AggregateConfigurationRejected"=2161770496, "Bad_TooManyMonitoredItems"=2161836032]  # OPC UA Subscription Service Status
        w274 = T6 refnum  # OPC UA client refnum
        w275 = refnum<event-registration> refnum  # OPC UA Data Change Event Registration Refnum
        n97 = Bundle(cluster=w268, "OPC UA Data Change Event Registration Refnum"=w275, "OPC UA client refnum"=w274, "OPC UA Subscription Service Status"=w273, "OPC UA Subscription ID"=w272, "OPC UA Monitored Nodes"=w271, "Connection Status"=w270) -> (w269:T13)
      }
      frame "Connect" {
        w277 = T14 ["s=Temperature", "s=fm40", "s=fm30", "s=wt20", "s=fm20", "s=fm60", "s=desiredPower", "s=bt11", "s=st10", "s=cx101", "s=at01", "s=powerInputSignal", "s=powerOutput", "s=flowData", "s=time", "s=bt41", "i=20001", "s=bt12", "s=bt21", "s=bt23", "s=bt25", "s=bt27", "s=bt29", "s=bt30", "s=bt32", "s=bt34", "s=bt43", "s=bt60", "s=bt63", "s=bt65", "s=bt66", "s=cx102", "s=cx103", "s=cx104", "s=cx111", "s=cx112", "s=cx113", "s=cx114", "s=st11", "s=st12n", "s=st12se", "s=st12sw", "s=st13", "s=st14e", "s=st14n", "s=st14s", "s=st14w", "s=wt13", "s=wt20", "s=wt22", "s=wt24", "s=wt26", "s=wt28", "s=wt31", "s=wt33", "s=wt35", "s=wt40", "s=wt42", "s=wt61", "s=wt62", "s=wt64", "s=wt67", "s=ctahFrequency", "s=pumpFrequency", "s=selectOperationMode", "s=tchxFrequency", "s=at02"] ("node IDs")
        n98 = call <vilib>:"Connect.vi"("trust any server (F)"=TRUE, "error in (no error)"=w285, "security policy"=T5 {"message mode"=enum."None", "security"=enum."Basic256"}, "server endpoint URL"="opc.tcp://18.119.107.49:4840") -> ("error out"=w292:errorcluster, "OPC UA client refnum out"=w288:T6)  [unwired: 5 in, 1 out]
        n99 = call <vilib>:"Create Subscription.vi"("error in (no error)"=w292, "publishing interval (1000 ms)"=10.0, "OPC UA client refnum in"=w288) -> ("error out"=w293:errorcluster, "OPC UA data change event"=w295:refnum<user-event>, "subscription ID out"=w289:T12, "OPC UA client refnum out"=w294:T6)  [unwired: 4 in, 1 out]
        n100 = call <vilib>:"Add Monitored Data Nodes.vi"("error in (no error)"=w293, "node IDs"=w277, "subscription ID in"=w289, "OPC UA client refnum in"=w294) -> ("error out"=w279:errorcluster, "OPC UA client refnum out"=w290:T6)  [unwired: 4 in, 2 out]
        n101 = register-events(w295) -> (reference out=w291:refnum<event-registration>)  [unwired: 2 in, 1 out]
        n102 = Bundle By Name(cluster=w281, "OPC UA Monitored Nodes"=w277, "OPC UA Data Change Event Registration Refnum"=w291, "OPC UA client refnum"=w290, "OPC UA Subscription ID"=w289, "Connection Status"=TRUE) -> (w278:T13)
      }
      frame "Stop Check" {
        n103 = Unbundle By Name(w298) -> ("Connection Status"=w297:bool)
        n104 = case shown="True" w297 {
          tunnel: ["Stop" w305] -> w300
          frame False {
          }
          frame True {
            n105 = Two Button Dialog(message="The Server is still connected. You will need to disconnect before stopping. Would you like to disconnect?", 1:"No" ("F button name (\"Cancel\")"), 2:"Yes" ("T button name (\"OK\")")) -> (T button?=w303:bool)
            n106 = case shown="True" w303 {
              tunnel: ["Standby" "Disconnect and Stop"] -> w305
              frame False {
              }
              frame True {
              }
            }
          }
        }
      }
      frame "Disconnect" {
        n107 = Unbundle By Name(w312) -> ("OPC UA Monitored Nodes"=w324:string[], "OPC UA client refnum"=w323:T6, "OPC UA Subscription ID"=w322:T12)
        n108 = Bundle By Name(cluster=w312, "Connection Status"=FALSE) -> (w311:T13)
        n109 = call <vilib>:"Delete Monitored Nodes.vi"("error in (no error)"=w318, "node IDs"=w324, "subscription ID in"=w322, "OPC UA client refnum in"=w323) -> ("error out"=w317:errorcluster, "OPC UA client refnum out"=w320:T6)  [unwired: 3 in, 3 out]
        n110 = Build Array(w322) -> (w321:T12[])
        n111 = call <vilib>:"Delete Subscriptions.vi"("error in (no error)"=w317, "subscription IDs"=w321, "OPC UA client refnum in"=w320) -> ("error out"=w316:errorcluster, "OPC UA client refnum out"=w319:T6)  [unwired: 6 in, 1 out]
        n112 = call <vilib>:"Disconnect.vi"("error in (no error)"=w316, "OPC UA client refnum in"=w319) -> ("error out"=w313:errorcluster)  [unwired: 9 in]
      }
      frame "Disconnect and Stop" {
        n113 = Unbundle By Name(w327) -> ("OPC UA Monitored Nodes"=w339:string[], "OPC UA client refnum"=w338:T6, "OPC UA Subscription ID"=w337:T12)
        n114 = Bundle By Name(cluster=w327, "Connection Status"=FALSE) -> (w326:T13)
        n115 = call <vilib>:"Delete Monitored Nodes.vi"("error in (no error)"=w333, "node IDs"=w339, "subscription ID in"=w337, "OPC UA client refnum in"=w338) -> ("error out"=w332:errorcluster, "OPC UA client refnum out"=w335:T6)  [unwired: 3 in, 3 out]
        n116 = Build Array(w337) -> (w336:T12[])
        n117 = call <vilib>:"Delete Subscriptions.vi"("error in (no error)"=w332, "subscription IDs"=w336, "OPC UA client refnum in"=w335) -> ("error out"=w331:errorcluster, "OPC UA client refnum out"=w334:T6)  [unwired: 6 in, 1 out]
        n118 = call <vilib>:"Disconnect.vi"("error in (no error)"=w331, "OPC UA client refnum in"=w334) -> ("error out"=w328:errorcluster)  [unwired: 9 in]
      }
      frame "Stop" {
      }
    }
    n119 = call "DAQ (SubVI).vi"("error in (no error)"=w5) -> ("error out"=→"error out":errorcluster, "Number of Disconnections"=→"Number of Disconnections":u32, "Available Elements for Reading"=→"Available Elements for Reading":i32, "DAQ?"=→"DAQ?":bool)  [unwired: 7 in]
    n120 = Or(x=w19, y=w17) -> (x .or. y?=w18:bool)
    n121 = Wait (ms)(milliseconds to wait=w11) -> (millisecond timer value=w10:u32)
  }
  n122 = call <vilib>:"Simple Error Handler.vi"("error in (no error)"=w3) -> ()  [unwired: 4 in, 5 out]
